vi "Configure Device.vi"(8 "error in (no error)":errorcluster, 10 "Max beams":dbl, 11 "NI DAQmx in":refnum<class "NI DAQmx.lvclass">) -> (0 "error out":errorcluster, 3 "NI DAQmx out":refnum<class "NI DAQmx.lvclass">)   [LabVIEW 2020, in "NI DAQmx.lvclass"]
uses:
  NI DAQmx.lvclass
  Controls/DAQmx line name.ctl
panel:
  in  "DAQmx line names":T1[](array[typedef])
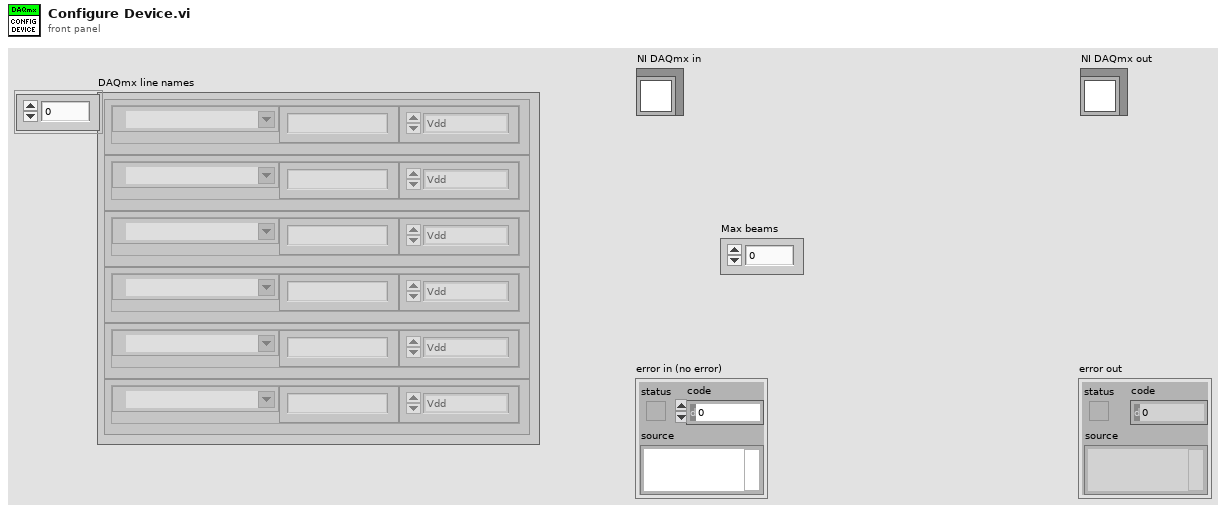
[diagram p1: front panel]
types:
  T1 = typedef "NI DAQmx.lvclass/DAQmx line name.ctl" = cluster{"lines":tag, "Function":string, "Function":enum16{"Vdd", "Control 0", "Control 1", "Control 2", "Control 3"}}
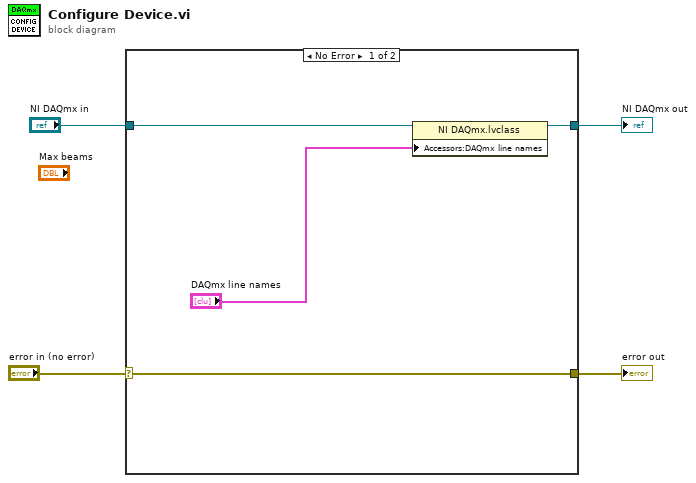
[diagram p0: block diagram]
diagram:
  n1 = case shown="No Error" "error in (no error)" {
    selector: "error in (no error)" -> [w6 w10]
    tunnel: [w6 w10] -> w3
    tunnel: [w7 w9] -> w2
    tunnel: "NI DAQmx in" -> [w8 w9]
    frame No Error {
      n2 = property class="NI DAQmx.lvclass"(reference=w8, "Accessors:DAQmx line names"="DAQmx line names") -> (reference out=w7:refnum<class "NI DAQmx.lvclass">)  [unwired: 1 in, 1 out]
    }
    frame Error {
    }
  }
  "error out" <- w3
  "NI DAQmx out" <- w2
